vi "DSF.Engine.BuilderManager.Set Builders.vi"(10 "Builders":refnum<class "DSF.Engine.Builder.lvclass">[](array[class]), 11 "Builder Manager in":refnum<class "DSF.Engine.BuilderManager.lvclass">) -> (3 "Builder Manager out":refnum<class "DSF.Engine.BuilderManager.lvclass">)   [LabVIEW 2017, in "DSF.Engine.lvlib" / "DSF.Engine.BuilderManager.lvclass"]
uses:
  DSF.Engine.BuilderManager.lvclass
  Builder/DSF.Engine.Builder.lvclass
  DSF.Engine.BuilderManager.lvclass/DSF.Engine.BuilderManager.ctl
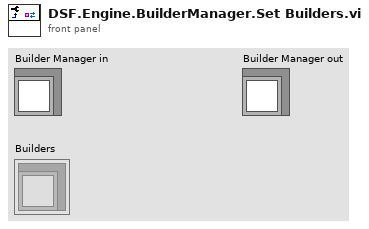
[diagram p1: front panel]
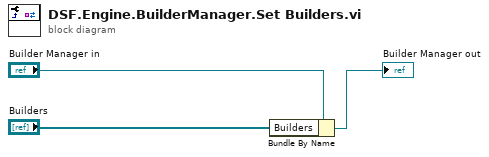
[diagram p0: block diagram]
diagram:
  n1 = Bundle By Name(cluster="Builder Manager in", "Builders"="Builders") -> (→"Builder Manager out":refnum<class "DSF.Engine.BuilderManager.lvclass">)
